vi "SetName.vi"(8 "error in":errorcluster, 10 "Name":string, 11 "camera.nit in":refnum<class "camera.lvclass">) -> (0 "error out":errorcluster)   [LabVIEW 2020, in "camera.lvclass"]
uses:
  camera.lvclass
  camera.lvclass/camera.ctl
  becbdec6-382f-4208-8a6a-87c009417815.vi
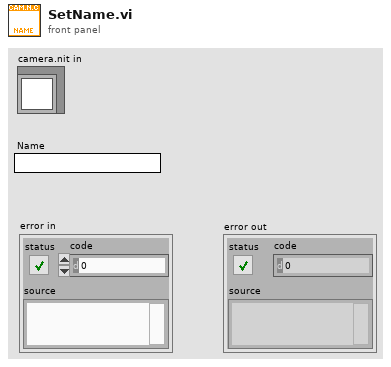
[diagram p1: front panel]
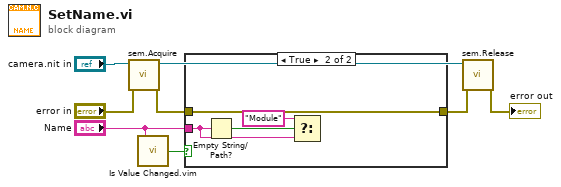
[diagram p0: block diagram]
diagram:
  n1 = call "sem.Acquire.vi"("error in"="error in", "camera.nit in"="camera.nit in") -> ("error out"=w3:errorcluster)  [unwired: 9 in]
  n2 = call "Is Value Changed.vim"("value"="Name") -> ("changed or first call?"=w2:bool)
  n3 = case shown="True" w2 {
    tunnel: [w8 w9] -> w5
    tunnel: w3 -> [w8 w9]
    tunnel: "Name" -> [_ w10]
    frame False {
    }
    frame True {
      n4 = Empty String/Path?(string/path=w10) -> (empty?=w11:bool)
      n5 = Select(t="Module", s=w11, f=w10) -> ()  [unwired: 1 out]
    }
  }
  n6 = call "sem.Release.vi"("error in"=w5, "camera.nit in"="camera.nit in") -> ("error out"=→"error out":errorcluster)  [unwired: 9 in]
